vi "generador de funciones.vi"() -> ()   [LabVIEW 2016]
panel:
  out "Waveform Chart":dbl(graph)
  in  "Enum":T1(ring)
  in  "Stop Button":bool
  out "Numeric Control":dbl
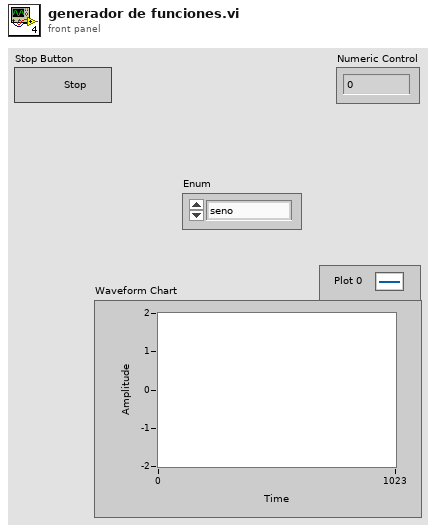
[diagram p1: front panel]
types:
  T1 = enum16{"seno", "pulso", "diente de sierra", "triangular", "tangente", "dc", "gnd"}
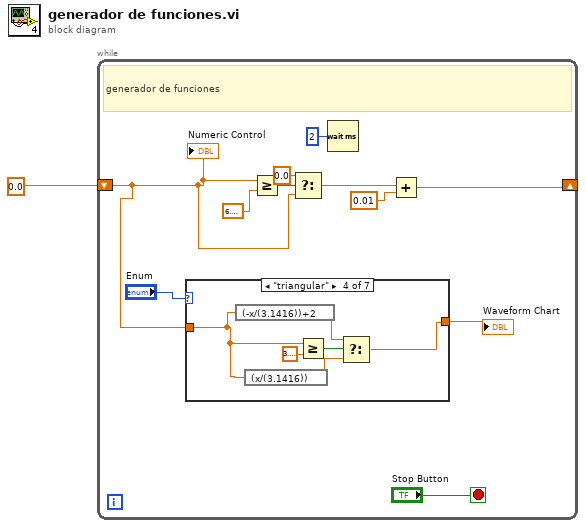
[diagram p0: block diagram]
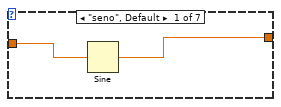
[diagram p2: hidden frame]
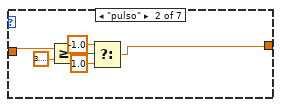
[diagram p3: hidden frame]
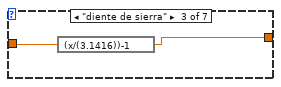
[diagram p4: hidden frame]
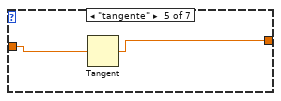
[diagram p5: hidden frame]
diagram:
  n1 = while {
    shift-right: [w12] -> _
    shift-left: 0.0 -> [w3]
    stop <- "Stop Button" stop-if-true
    # "generador de funciones"
    n2 = case shown="\"triangular\"" "Enum" {
      tunnel: w3 -> [w14 w20 w22 w25 w29 _ _]
      tunnel: [w13 w15 w21 w26 w30 _ _] -> w2
      frame "seno", Default {
        n3 = Sine(x=w14) -> (sin(x)=w13:dbl)
      }
      frame "pulso" {
        n4 = Greater Or Equal?(x=w20, y=3.141592653589793) -> (x >= y?=w18:bool)
        n5 = Select(t=-1.0, s=w18, f=1.0) -> (s? t:f=w15:dbl)
      }
      frame "diente de sierra" {
        n6 = expression code="(x/(3.1416))-1"(w22) -> (w21:dbl)
      }
      frame "triangular" {
        n7 = expression code="(-x/(3.1416))+2"(w25) -> (w24:dbl)
        n8 = expression code="(x/(3.1416))"(w25) -> (w23:dbl)
        n9 = Greater Or Equal?(x=w25, y=3.141592653589793) -> (x >= y?=w27:bool)
        n10 = Select(t=w24, s=w27, f=w23) -> (s? t:f=w26:dbl)
      }
      frame "tangente" {
        n11 = Tangent(1:w29) -> (0:w30:dbl)
      }
      frame "dc" {
      }
      frame "gnd" {
      }
    }
    "Waveform Chart" <- w2
    n12 = Greater Or Equal?(x=w3, y=6.283185307179586) -> (x >= y?=w7:bool)
    n13 = Select(t=0.0, s=w7, f=w3) -> (s? t:f=w5:dbl)
    n14 = Wait (ms)(milliseconds to wait=u32 2) -> ()  [unwired: 1 out]
    n15 = Add(x=w5, y=0.01) -> (x+y=w12:dbl)
    "Numeric Control" <- w3
  }
